vi "NK11003_Read.vi"(8 "error in":errorcluster caption="错误输入（无错误）", 11 "MyIndex":u8) -> (0 "error out":errorcluster caption="错误输出", 2 "电流":dbl, 3 "电压":dbl)   [LabVIEW 2015]
uses:
  <vilib>/Instr/_visa.llb/VISA Configure Serial Port (Instr).vi
panel:
  out "VISA":refnum<visa-resource-name> caption="VISA资源名称输出"
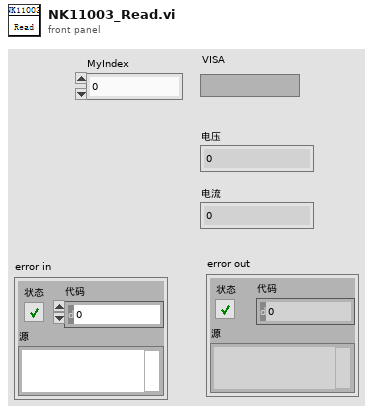
[diagram p1: front panel]
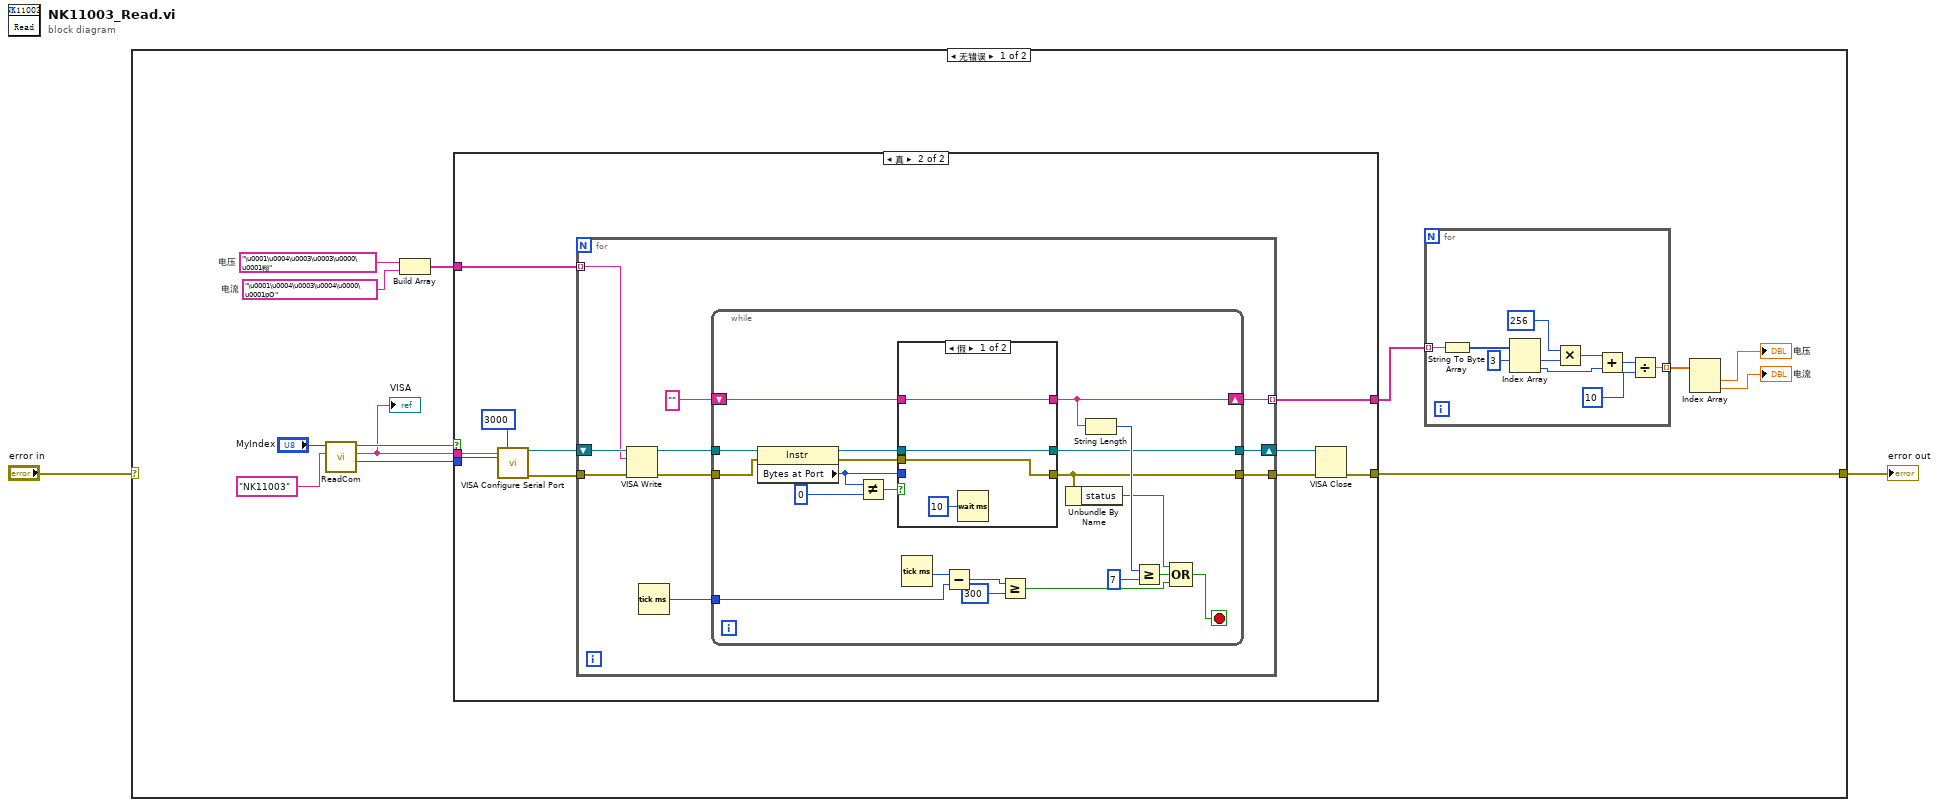
[diagram p0: block diagram]
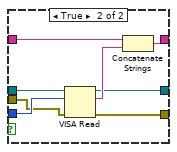
[diagram p3: hidden frame]
diagram:
  n1 = case shown="无错误" "error in" {
    selector: "error in" -> [_ w79]
    tunnel: [w3 w79] -> w1
    frame No Error {
      w12 = "\u0001\u0004\u0003\u0004\u0000\u0001pO"  # 电流
      w14 = "\u0001\u0004\u0003\u0003\u0000\u0001翈"  # 电压
      n2 = call "ReadCom.vi"("仪器名称"="NK11003", "MyIndex"="MyIndex") -> ("Baudrate"=w5:i32, "COM"=w4:string, "OK?"=w6:bool)  [unwired: 7 in]
      "VISA" <- w4
      n3 = Build Array(w14, w12) -> (w13:string[])
      n4 = case shown="真" w6 {
        tunnel: [_ w21] -> w15
        tunnel: w13 -> [_ w20]
        tunnel: w4 -> [_ w19]
        tunnel: w5 -> [_ w17]
        tunnel: [_ w16] -> w3
        frame False {
        }
        frame True {
          n5 = call-poly "VISA Configure Serial Port"("VISA resource name"=w19, "timeout (10sec)"=u32 3000, "baud rate (9600)"=w17) -> ("VISA resource name out"=w25:refnum<visa-resource-name>, "error out"=w24:errorcluster)  [unwired: 11 in]
          n6 = for {
            tunnel: w20 -> [w27] mode=indexing
            shift-right: [w29] -> w23
            shift-left: w25 -> [w35]
            tunnel: w24 -> [w34]
            tunnel: [w26] -> w22
            tunnel: [w28] -> w21 mode=indexing
            n7 = VISA Write(VISA resource name=w35, write buffer=w27, error in (no error)=w34) -> (VISA resource name out=w32:refnum<visa-resource-name>, error out=w33:errorcluster)  [unwired: 1 out]
            n8 = Tick Count (ms)() -> (millisecond timer value=w30:u32)
            n9 = while {
              tunnel: w33 -> [w36]
              tunnel: w32 -> [w56]
              shift-right: [w49] -> w28
              shift-left: "" -> [w50]
              tunnel: w30 -> [w42]
              tunnel: [w38] -> w29
              tunnel: [w37] -> w26
              stop <- w45 stop-if-true
              n10 = property class="Instr"(reference=w56, error in=w36) -> (reference out=w53:refnum<visa-resource-name>, error out=w51:errorcluster, "Bytes at Port"=w52:u32)
              n11 = Not Equal?(x=w52, y=u32 0) -> (x != y?=w54:bool)
              n12 = case shown="假" w54 {
                tunnel: w53 -> [w57 w68]
                tunnel: w52 -> [_ w67]
                tunnel: w51 -> [w58 w66]
                tunnel: w50 -> [w59 w65]
                tunnel: [w59 w63] -> w49
                tunnel: [w58 w62] -> w37
                tunnel: [w57 w61] -> w38
                frame False {
                  n13 = Wait (ms)(milliseconds to wait=u32 10 ("等待时间（毫秒）")) -> ()  [unwired: 1 out]
                }
                frame True {
                  n14 = VISA Read(VISA resource name=w68, byte count=w67, error in (no error)=w66) -> (VISA resource name out=w61:refnum<visa-resource-name>, read buffer=w64:string, error out=w62:errorcluster)  [unwired: 1 out]
                  n15 = Concatenate Strings(w65, w64) -> (w63:string)
                }
              }
              n16 = Tick Count (ms)() -> (millisecond timer value=w43:u32)
              n17 = Subtract(x=w43, y=w42) -> (x-y=w41:u32)
              n18 = Greater Or Equal?(x=w41, y=u32 300) -> (x >= y?=w39:bool)
              n19 = Unbundle By Name(w37) -> ("status"=w44:bool)
              n20 = String Length(string=w49) -> (length=w48:i32)
              n21 = Greater Or Equal?(x=w48, y=7) -> (x >= y?=w47:bool)
              n22 = Compound Arithmetic op=OR ("复合运算")(w44, w47, w39) -> (w45:bool)
            }
          }
          n23 = VISA Close(VISA resource name=w23, error in (no error)=w22) -> (error out=w16:errorcluster)
        }
      }
      n24 = for {
        tunnel: w15 -> [w70] mode=indexing
        tunnel: [w69] -> w11 mode=indexing
        n25 = String To Byte Array(string=w70) -> (unsigned byte array=w71:u8[])
        n26 = Index Array(array=w71, index #1=3 ("索引")) -> (element #1=w77:u8, element #2=w74:u8)  [unwired: 1 in]
        n27 = Multiply(x=u16 256 ("y"), y=w77) -> (x*y=w75:u16)
        n28 = Add(x=w75, y=w74) -> (x+y=w73:u16)
        n29 = Divide(x=w73, y=u16 10) -> (x/y=w69:dbl)
      }
      n30 = Index Array(array=w11) -> (element #1=→"电压":dbl, element #2=→"电流":dbl)  [unwired: 2 in]
    }
    frame Error {
    }
  }
  "error out" <- w1
